vi "Handle.vi"(11 "Dev Actor in":refnum<class "Dev Actor.lvclass">) -> (2 "Destroy?":bool, 3 "Dev Actor out":refnum<class "Dev Actor.lvclass">)   [LabVIEW 2021, in "Dev Actor.lvlib" / "Dev Actor.lvclass"]
uses:
  Dev Actor.lvclass
  Dev Actor.lvclass/Dev Actor.ctl
  <vilib>/jettl/jettl/Actor/Actor/Actor.lvclass
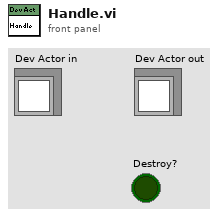
[diagram p1: front panel]
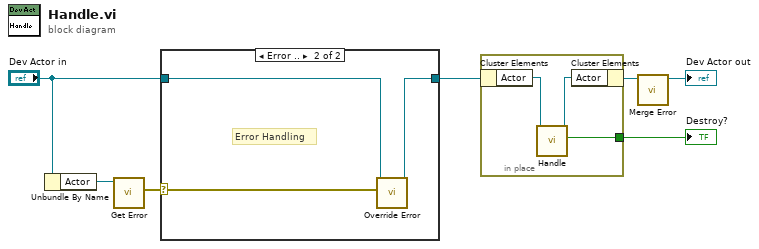
[diagram p0: block diagram]
diagram:
  n1 = Unbundle By Name("Dev Actor in") -> ("Actor"=w5:refnum<class "Actor.lvclass">)
  n2 = call-dynamic "Get Error.vi"("Actor in"=w5) -> ("Error"=w6:errorcluster)  [unwired: 10 in]
  n3 = case shown="Error .." w6 {
    selector: w6 -> [_ w9]
    tunnel: "Dev Actor in" -> [w8 w11]
    tunnel: [w8 w10] -> w2
    frame No Error {
    }
    frame Error {
      # "Error Handling"
      n4 = call-dynamic "Override Error.vi"("Error"=w9, "Dev Actor in"=w11) -> ("Dev Actor out"=w10:refnum<class "Dev Actor.lvclass">)  [unwired: 9 in]
    }
  }
  n5 = in-place {
    in-place-border: [w12] -> w1
    n6 = in-place-cluster #1(w2) -> ("Actor"=w14:refnum<class "Actor.lvclass">)
    n7 = call-dynamic "Handle.vi"("Actor in"=w14) -> ("Destroy?"=w12:bool, "Actor out"=w13:refnum<class "Actor.lvclass">)  [unwired: 9 in]
    n8 = in-place-cluster #1("Actor"=w13) -> (w4:refnum<class "Dev Actor.lvclass">)
  }
  "Destroy?" <- w1
  n9 = call-dynamic "Merge Error.vi"("Dev Actor in"=w4) -> ("Dev Actor out"=→"Dev Actor out":refnum<class "Dev Actor.lvclass">)  [unwired: 10 in]
